vi "Filter 2D array by column names.vi"(10 "Array in":string[][](array[string]), 11 "Array 3":string[](array[string])) -> (3 "Array out":string[][](array[string]))   [LabVIEW 2013]
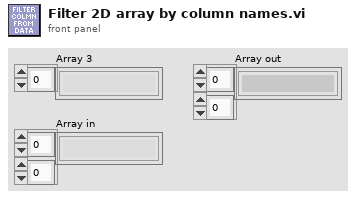
[diagram p1: front panel]
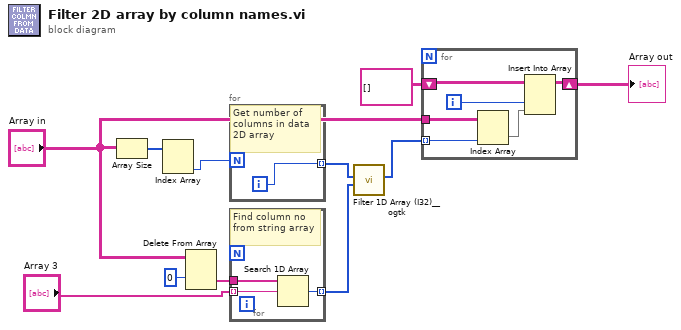
[diagram p0: block diagram]
diagram:
  n1 = Array Size(array="Array in") -> (size(s)=w6:i32[])
  n2 = Index Array(array=w6) -> (element #2=w7:i32)  [unwired: 2 in, 1 out]
  n3 = Delete From Array(array="Array in", index (row)=0) -> (deleted portion=w2:string[])  [unwired: 2 in, 1 out]
  n4 = for {
    N: w7 -> [_]
    tunnel: [w12] -> w10 mode=indexing
    i -> [w12]
    # "Get number of columns in data 2D array"
  }
  n5 = for {
    tunnel: w2 -> [w15]
    tunnel: "Array 3" -> [w14] mode=indexing
    tunnel: [w13] -> w9 mode=indexing
    # "Find column no from string array"
    n6 = Search 1D Array(1D array=w15, element=w14) -> (index of element=w13:i32)  [unwired: 1 in]
  }
  n7 = call "Filter 1D Array (I32)__ogtk.vi"("items to filter"=w9, "array"=w10) -> ("filtered array"=w11:i32[])  [unwired: 4 in, 1 out]
  n8 = for {
    shift-right: [w19] -> w8
    shift-left: string[][] [] -> [w20]
    tunnel: "Array in" -> [w21]
    tunnel: w11 -> [w16] mode=indexing
    i -> [w18]
    n9 = Index Array(array=w21, index (col)=w16) -> (element=w17:string[])  [unwired: 1 in]
    n10 = Insert Into Array(array=w20, index (col)=w18, new element=w17) -> (w19:string[][])  [unwired: 1 in]
  }
  "Array out" <- w8
